vi "2 WaypointHeadingGoodness.vi"(3 "Waypoint Location":T2 {"North" format="%#_10f"; "East" format="%#_8f"}, 4 "Heading\nto Test":T1 format="%05.1f") -> (1 "Goodness":dbl)   [LabVIEW 2011]
doc: "Takes the absolute wind vector, the heading of your next waypoint, and a test heading and outputs a goodness value for the test heading. The criteria is the speed to get to the waypoint.\n\nThe goodness is evaluated by taking the softmax of an angle with all possible complimenting angles (i.e. if the test heading is 10 degrees it is matched with -1 through -89; note that angles are adjusted to be degrees from directly at the waypoint). The specific calculation for finding the net velocity of a pair of angles requires the velocities from the polar plot."
uses:
  2 Typedefs/UTM Location.ctl
  2 Typedefs/heading.ctl
  2 Globals/2 Global.vi
  2 Globals/2 TuningConstants.vi
panel:
  out "Heading to Waypt":dbl
  # "Inputs"
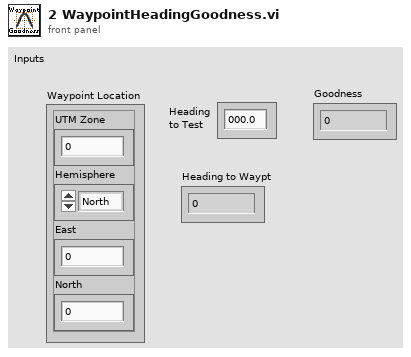
[diagram p1: front panel]
types:
  T1 = typedef "heading.ctl" = dbl
  T2 = typedef "UTM Location.ctl" = cluster{"UTM Zone":dbl, "Hemisphere":enum16{"North", "South"}, "East":dbl, "North":dbl}
  T3 = typedef "absolute wind direction.ctl" = dbl
  T4 = typedef "absolute wind speed.ctl" = dbl
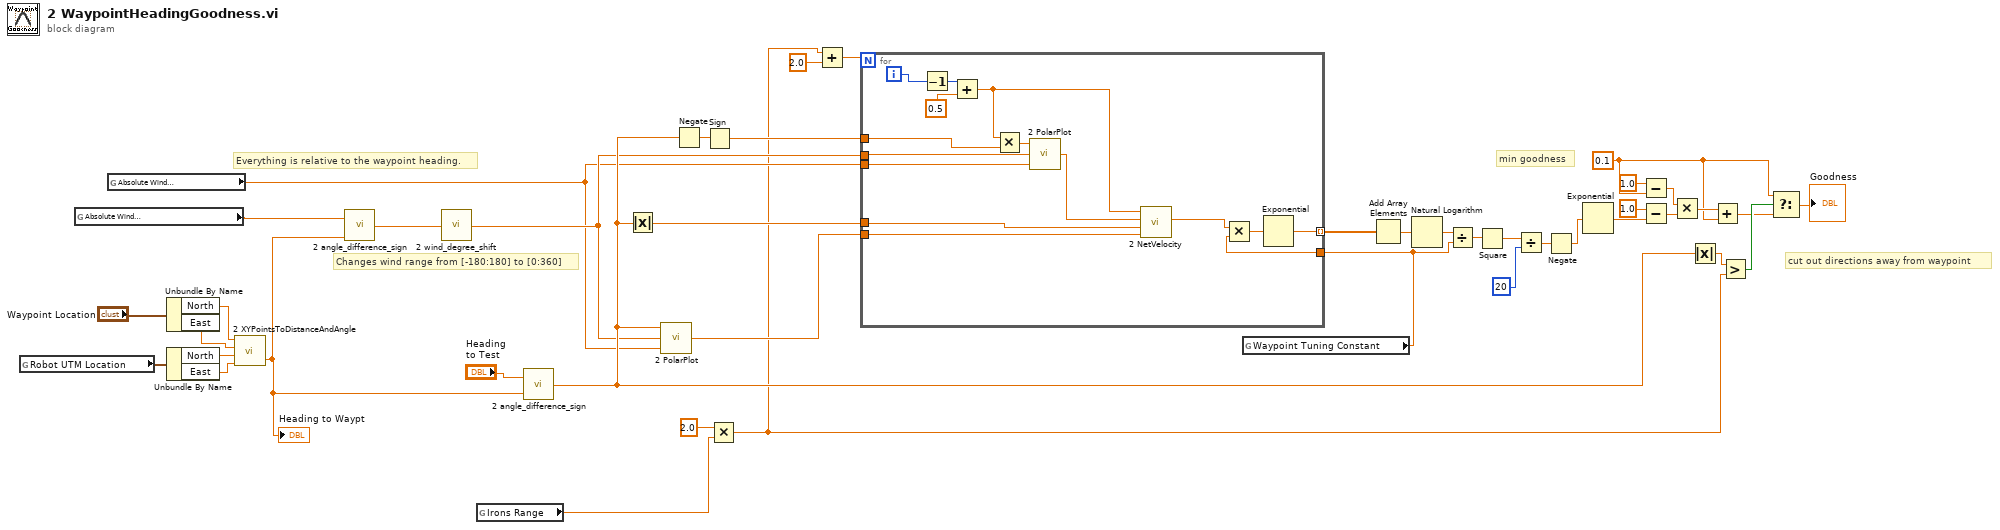
[diagram p0: block diagram]
diagram:
  w7 = 0.1
  # "cut out directions away from waypoint"
  # "min goodness"
  # "Changes wind range from [-180:180] to [0:360]"
  # "Everything is relative to the waypoint heading."
  n1 = global read "2 Global.vi" "Robot UTM Location"() -> (w23:T2)
  n2 = global read "2 Global.vi" "Absolute Wind\nDirection (º)"() -> (w12:T3)
  n3 = global read "2 Global.vi" "Absolute Wind\nSpeed"() -> (w13:T4)
  n4 = Unbundle By Name("Waypoint Location") -> ("North"=w32:dbl, "East"=w31:dbl)
  n5 = Unbundle By Name(w23) -> ("North"=w33:dbl, "East"=w34:dbl)
  n6 = call "2 XYPointsToDistanceAndAngle.vi"("East 2"=w34, "North 2"=w33, "East 1"=w31, "North 1"=w32) -> ("Angle Diff"=w41:dbl)  [unwired: 1 out]
  "Heading to Waypt" <- w41
  n7 = call "2 angle_difference_sign.vi"("Angle 2"=w41, "Angle 1"=w12) -> ("Difference"=w42:dbl)
  n8 = call "2 wind_degree_shift.vi"("Wind Theta -180 - 180"=w42) -> ("Wind Theta 0-360"=w14:dbl)
  n9 = global read "2 TuningConstants.vi" "Irons Range"() -> (w5:dbl)
  n10 = call "2 angle_difference_sign.vi"("Angle 2"=w41, "Angle 1"="Heading\nto Test") -> ("Difference"=w19:dbl)
  n11 = Absolute Value(x=w19) -> (abs(x)=w17:dbl)
  n12 = call "2 PolarPlot.vi"("Apparent Wind\nSpeed"=w13, "Apparent Wind\nDirection (º)"=w14, "Boat Angle"=w19) -> ("Velocity"=w16:dbl)
  n13 = Negate(x=w19) -> (-x=w20:dbl)
  n14 = Sign(1:w20) -> (0:w21:dbl)
  n15 = Multiply(x=2.0, y=w5) -> (x*y=w1:dbl)
  n16 = Add(x=w1, y=2.0) -> (x+y=w3:dbl)
  n17 = global read "2 TuningConstants.vi" "Waypoint Tuning Constant"() -> (w18:dbl)
  n18 = for {
    N: w3 -> [_]
    tunnel: [w55] -> w24 mode=indexing
    tunnel: w21 -> [w46]
    tunnel: w18 -> [w50]
    tunnel: w17 -> [w52]
    tunnel: w16 -> [w51]
    tunnel: w13 -> [w47]
    tunnel: w14 -> [w45]
    i -> [w43]
    n19 = Decrement(x=w43) -> (x-1=w44:i32)
    n20 = Add(x=w44, y=0.5) -> (x+y=w48:dbl)
    n21 = Multiply(x=w48, y=w46) -> (x*y=w57:dbl)
    n22 = call "2 PolarPlot.vi"("Apparent Wind\nSpeed"=w47, "Apparent Wind\nDirection (º)"=w45, "Boat Angle"=w57) -> ("Velocity"=w53:dbl)
    n23 = call "2 NetVelocity.vi"("Speed 2"=w51, "Angle 2"=w52, "Speed 1"=w53, "Angle 1"=w48) -> ("Net Velocity"=w49:dbl)  [unwired: 7 in]
    n24 = Multiply(x=w49, y=w50) -> (x*y=w54:dbl)
    n25 = Exponential(1:w54) -> (0:w55:dbl)
  }
  n26 = Add Array Elements(numeric array=w24) -> (sum=w27:dbl)
  n27 = Natural Logarithm(1:w27) -> (0:w26:dbl)
  n28 = Divide(x=w26, y=w18) -> (x/y=w25:dbl)
  n29 = Square(x=w25) -> (x^2=w28:dbl)
  n30 = Divide(x=w28, y=20) -> (x/y=w29:dbl)
  n31 = Negate(x=w29) -> (-x=w36:dbl)
  n32 = Exponential(1:w36) -> (0:w37:dbl)
  n33 = Subtract(x=1.0, y=w7) -> (x-y=w9:dbl)
  n34 = Subtract(x=1.0, y=w37) -> (x-y=w11:dbl)
  n35 = Multiply(x=w9, y=w11) -> (x*y=w8:dbl)
  n36 = Absolute Value(x=w19) -> (abs(x)=w39:dbl)
  n37 = Add(x=w8, y=w7) -> (x+y=w6:dbl)
  n38 = Greater?(x=w39, y=w1) -> (0:w40:bool)
  n39 = Select(t=w7, s=w40, f=w6) -> (s? t:f=→"Goodness":dbl)
